vi "Set Basic Pump Parameters 2 (SubVI).vi"(0 "Units":string, 1 "error out 2":errorcluster, 2 "Target Volume":dbl, 5 "Flow rate":dbl, 6 "Direction":string(combo), 7 "Pump Add":string, 8 "diameter (mm)":dbl, 9 "Send":bool, 10 "VISA resource name out 2":refnum<visa-resource-name>) -> (3 "VISA resource name out":refnum<visa-resource-name>, 4 "error out":errorcluster)   [LabVIEW 2020]
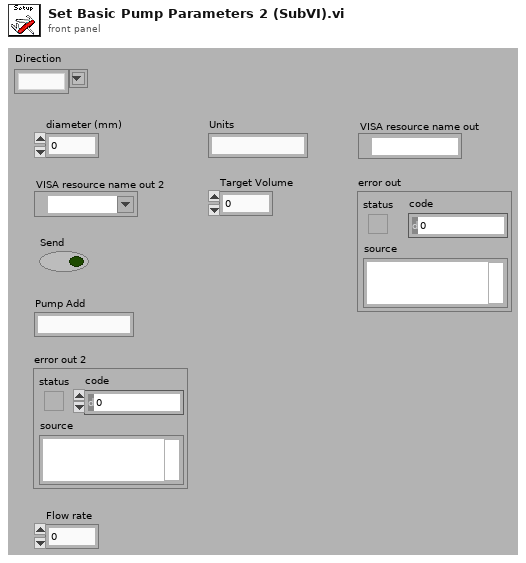
[diagram p1: front panel]
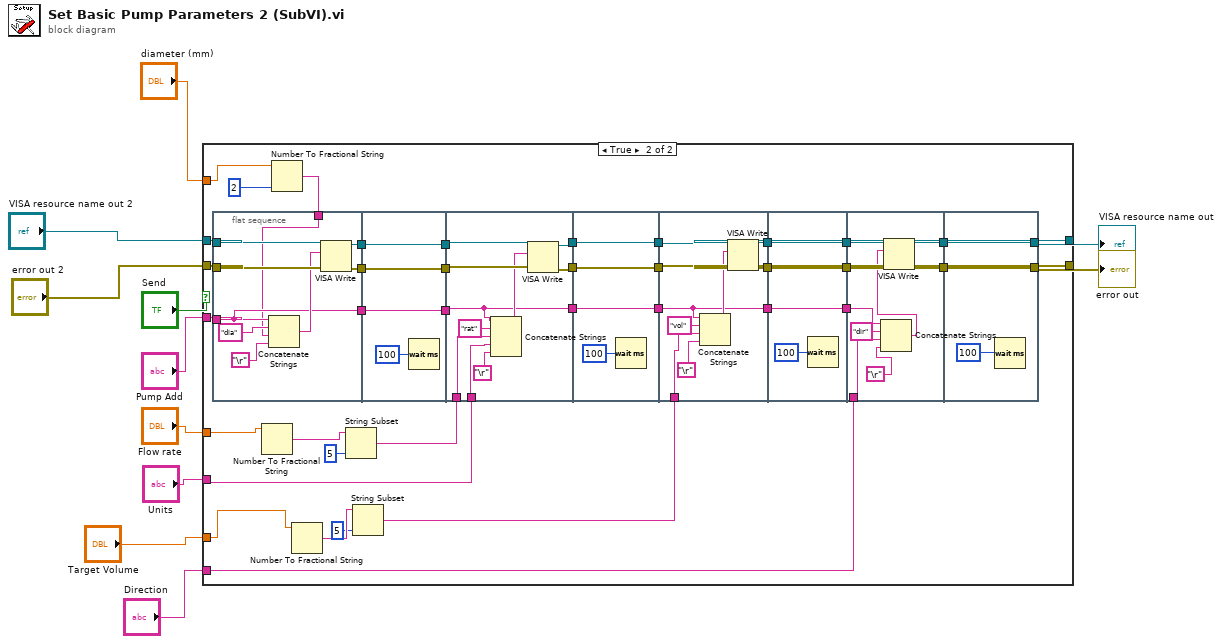
[diagram p0: block diagram]
diagram:
  n1 = case shown="True" "Send" {
    tunnel: "VISA resource name out 2" -> [w13 w51]
    tunnel: "error out 2" -> [w12 w50]
    tunnel: [w13 w49] -> w10
    tunnel: [w12 w48] -> w11
    tunnel: "Pump Add" -> [_ w47]
    tunnel: "diameter (mm)" -> [_ w17]
    tunnel: "Flow rate" -> [_ w18]
    tunnel: "Units" -> [_ w46]
    tunnel: "Target Volume" -> [_ w14]
    tunnel: "Direction" -> [_ w27]
    frame False {
    }
    frame True {
      n2 = flat-sequence {
        tunnel: w51 -> [w60]
        tunnel: w50 -> [w59]
        tunnel: [w58] -> w45
        tunnel: [w57] -> w43
        tunnel: w47 -> [w53]
        tunnel: [w53] -> w41
        tunnel: w16 -> [w52]
        tunnel: w45 -> [w64]
        tunnel: [w64] -> w44
        tunnel: w43 -> [w63]
        tunnel: [w63] -> w42
        tunnel: w41 -> [w62]
        tunnel: [w62] -> w40
        tunnel: w44 -> [w74]
        tunnel: w42 -> [w72]
        tunnel: w40 -> [w65]
        tunnel: w23 -> [w69]
        tunnel: w46 -> [w68]
        tunnel: [w73] -> w39
        tunnel: [w71] -> w37
        tunnel: [w65] -> w35
        tunnel: w39 -> [w78]
        tunnel: [w78] -> w38
        tunnel: w37 -> [w77]
        tunnel: [w77] -> w36
        tunnel: w35 -> [w76]
        tunnel: [w76] -> w34
        tunnel: w38 -> [w85]
        tunnel: w36 -> [w84]
        tunnel: w34 -> [w79]
        tunnel: w19 -> [w81]
        tunnel: [w86] -> w33
        tunnel: [w87] -> w32
        tunnel: [w79] -> w29
        tunnel: w33 -> [w91]
        tunnel: w32 -> [w90]
        tunnel: [w91] -> w31
        tunnel: [w90] -> w30
        tunnel: w29 -> [w88]
        tunnel: [w88] -> w28
        tunnel: w31 -> [w100]
        tunnel: w30 -> [w97]
        tunnel: w28 -> [w94]
        tunnel: w27 -> [w92]
        tunnel: [w99] -> w26
        tunnel: [w98] -> w25
        tunnel: [w102] -> w48
        tunnel: [w103] -> w49
        tunnel: w26 -> [w103]
        tunnel: w25 -> [w102]
        frame #0 {
          n3 = Concatenate Strings(w53, "dia" ("string"), w52, "\r") -> (w55:string)
          n4 = VISA Write(VISA resource name=w60, write buffer=w55, error in (no error)=w59) -> (VISA resource name out=w58:refnum<visa-resource-name>, error out=w57:errorcluster)  [unwired: 1 out]
        }
        frame #1 {
          n5 = Wait (ms)(milliseconds to wait=u32 100) -> ()  [unwired: 1 out]
        }
        frame #2 {
          n6 = Concatenate Strings(w65, "rat" ("string"), w69, w68, "\r") -> (w66:string)
          n7 = VISA Write(VISA resource name=w74, write buffer=w66, error in (no error)=w72) -> (VISA resource name out=w73:refnum<visa-resource-name>, error out=w71:errorcluster)  [unwired: 1 out]
        }
        frame #3 {
          n8 = Wait (ms)(milliseconds to wait=u32 100) -> ()  [unwired: 1 out]
        }
        frame #4 {
          n9 = Concatenate Strings(w79, "vol" ("string"), w81, "\r") -> (w80:string)
          n10 = VISA Write(VISA resource name=w85, write buffer=w80, error in (no error)=w84) -> (VISA resource name out=w86:refnum<visa-resource-name>, error out=w87:errorcluster)  [unwired: 1 out]
        }
        frame #5 {
          n11 = Wait (ms)(milliseconds to wait=u32 100) -> ()  [unwired: 1 out]
        }
        frame #6 {
          n12 = Concatenate Strings(w94, "dir" ("string"), w92, "\r") -> (w96:string)
          n13 = VISA Write(VISA resource name=w100, write buffer=w96, error in (no error)=w97) -> (VISA resource name out=w99:refnum<visa-resource-name>, error out=w98:errorcluster)  [unwired: 1 out]
        }
        frame #7 {
          n14 = Wait (ms)(milliseconds to wait=u32 100) -> ()  [unwired: 1 out]
        }
      }
      n15 = Number To Fractional String(number=w18) -> (F-format string=w22:string)  [unwired: 3 in]
      n16 = Number To Fractional String(number=w17, precision (6)=2) -> (F-format string=w16:string)  [unwired: 2 in]
      n17 = Number To Fractional String(number=w14) -> (F-format string=w21:string)  [unwired: 3 in]
      n18 = String Subset(string=w22, length (rest)=5 ("length (rest)")) -> (substring=w23:string)  [unwired: 1 in]
      n19 = String Subset(string=w21, length (rest)=5 ("length (rest)")) -> (substring=w19:string)  [unwired: 1 in]
    }
  }
  "error out" <- w11
  "VISA resource name out" <- w10
